vi "EXA_logEvent_DetailedState.vi"(8 "error in (no error)":errorcluster, 11 "logevent_DetailedState_Ctl":T1) -> (0 "error out":errorcluster, 2 "function return":i32, 3 "logevent_DetailedState_Ctl out":T1)   [LabVIEW 2016, in "SALLV_EXA.lvlib"]
doc: "int EXA_shm_logEvent_DetailedStateLV(EXA_logevent_DetailedStateLV *logevent_DetailedState_Ctl );"
uses:
  SALLV_EXA.lvlib
  DataTypes/logevent_DetailedState.ctl
  SALLV_EXA.so
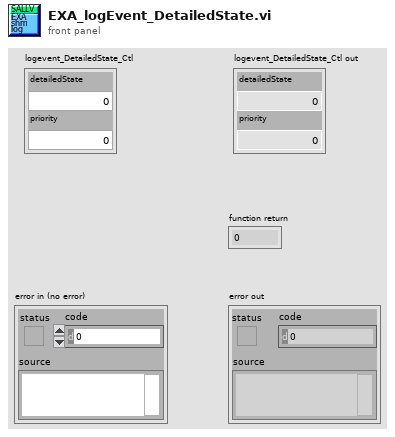
[diagram p1: front panel]
types:
  T1 = typedef "SALLV_EXA.lvlib/logevent_DetailedState.ctl" = cluster{"detailedState":u16, "priority":i32}
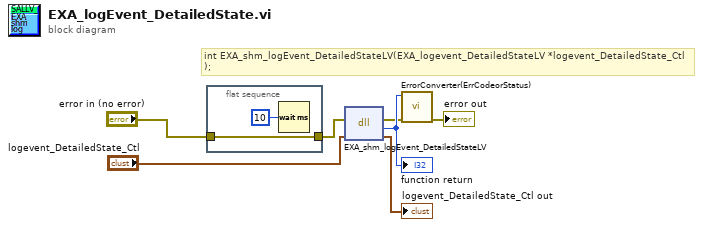
[diagram p0: block diagram]
diagram:
  # "int EXA_shm_logEvent_DetailedStateLV(EXA_logevent_DetailedStateLV *logevent_DetailedState_Ctl );"
  n1 = flat-sequence {
    tunnel: "error in (no error)" -> [w9]
    tunnel: [w9] -> w1
    frame #0 {
      n2 = Wait (ms)(milliseconds to wait=u32 10) -> ()  [unwired: 1 out]
    }
  }
  n3 = dll-call lib="home/andres/ct_cmpuserevents/ts_sallv_exa/SALLV_EXA.*" fn="EXA_shm_logEvent_DetailedStateLV"(error in=w1, "logevent_DetailedState_Ctl"="logevent_DetailedState_Ctl") -> (error out=w4:errorcluster, w7:i32, "logevent_DetailedState_Ctl"=→"logevent_DetailedState_Ctl out":T1)  [unwired: 2 in, 1 out]
  "function return" <- w7
  n4 = call "ErrorConverter(ErrCodeorStatus).vi"("error in (no error)"=w4, "error code"=w7) -> ("error out"=→"error out":errorcluster)  [unwired: 9 in]
